vi "S2C_FORNAX_Proc_Commands.vi"(7 "VI_Ref":refnum<vi>, 8 "Error In":errorcluster, 10 "Settings":T1, 11 "Q-Ref":refnum<queue>) -> (0 "Error Out":errorcluster, 2 "Exit?":bool, 3 "Response":variant)   [LabVIEW 2015]
uses:
  S2C_FORNAX_Proc_Globals.vi
panel:
  out "Ref":refnum<k5>
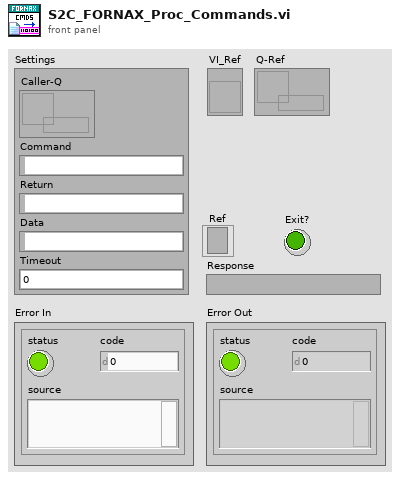
[diagram p1: front panel]
types:
  T1 = cluster{"Caller-Q":refnum<queue>, "Command":string, "Return":string, "Data":variant, "Timeout":dbl}
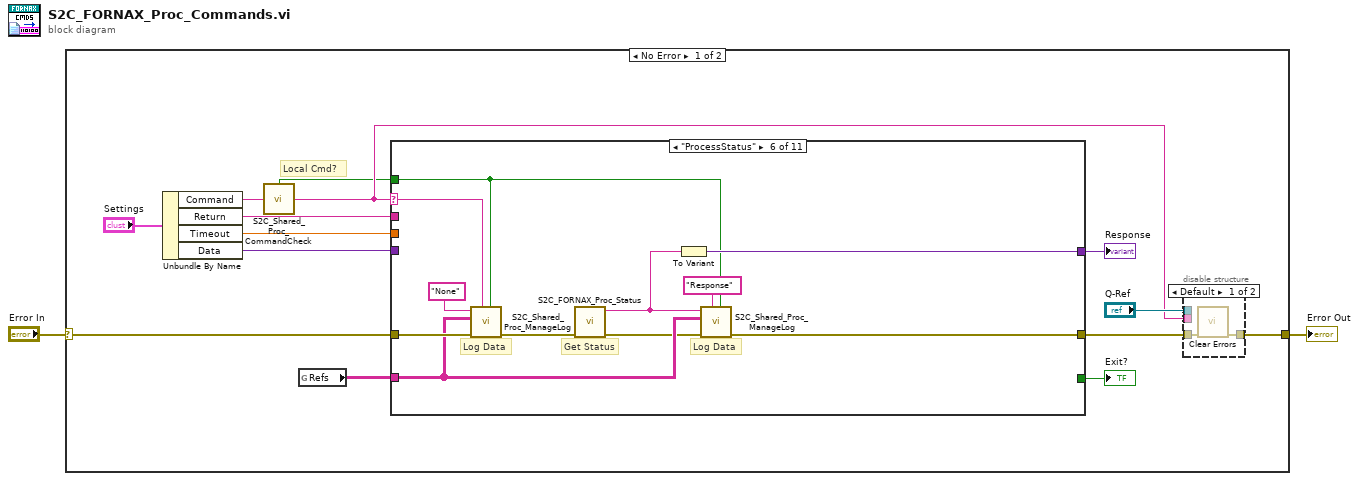
[diagram p0: block diagram]
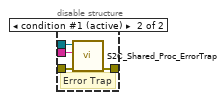
[diagram p2: hidden frame]
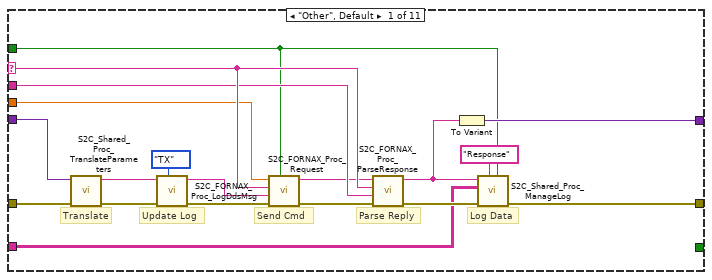
[diagram p3: hidden frame]
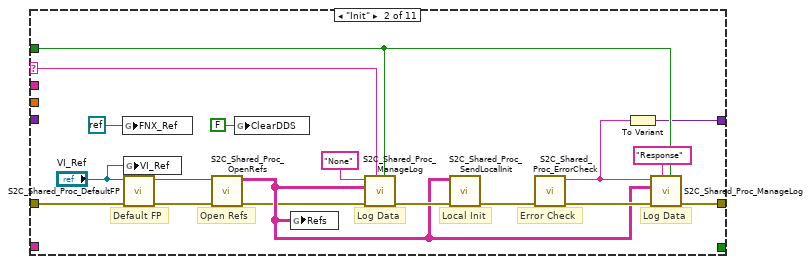
[diagram p4: hidden frame]
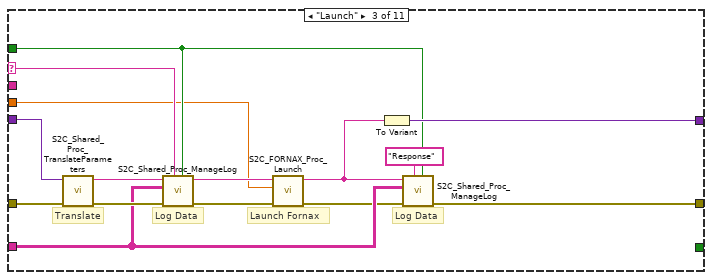
[diagram p5: hidden frame]
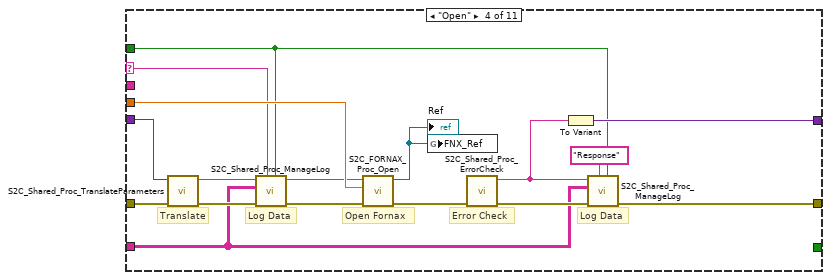
[diagram p6: hidden frame]
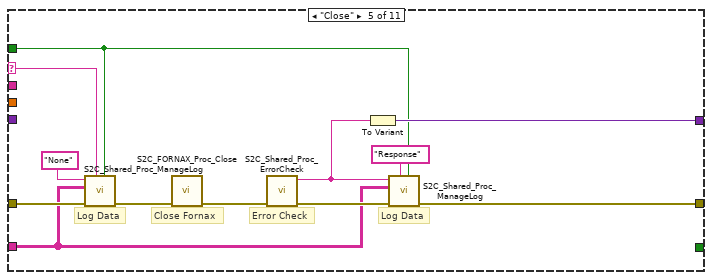
[diagram p7: hidden frame]
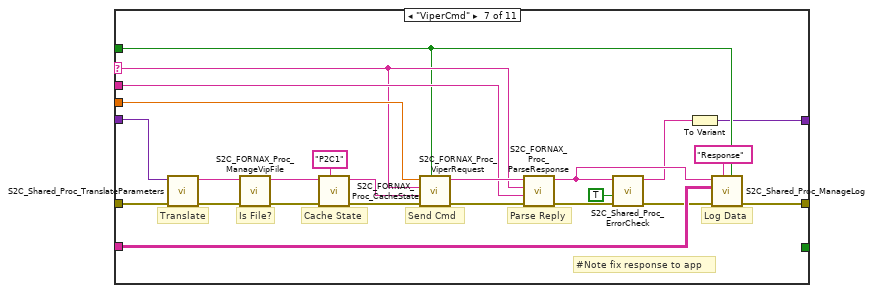
[diagram p8: hidden frame]
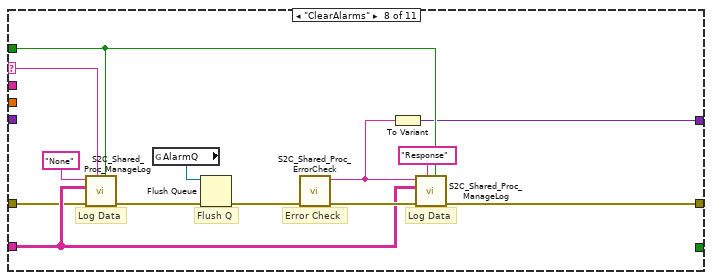
[diagram p9: hidden frame]
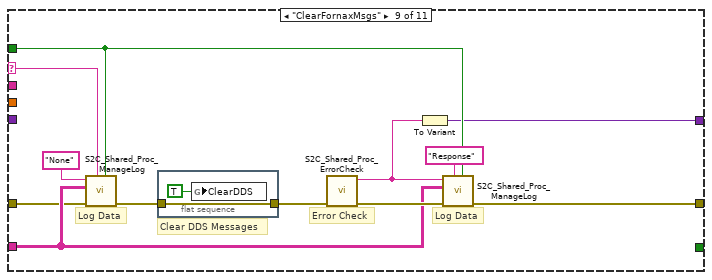
[diagram p10: hidden frame]
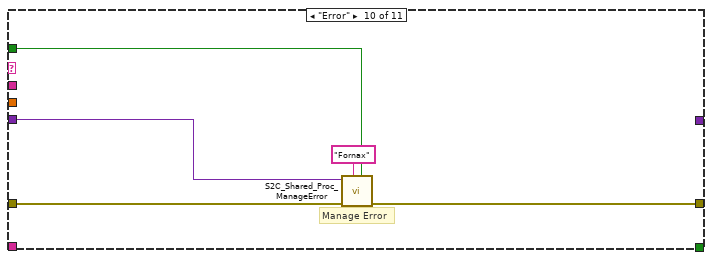
[diagram p11: hidden frame]
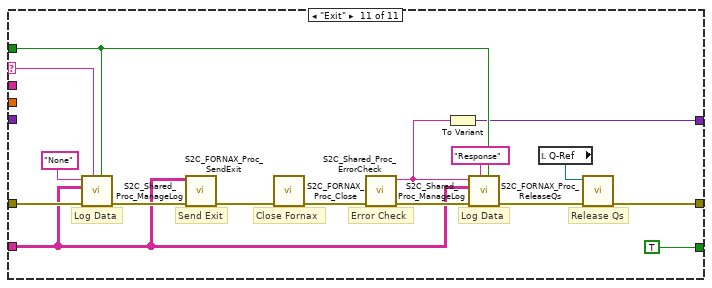
[diagram p12: hidden frame]
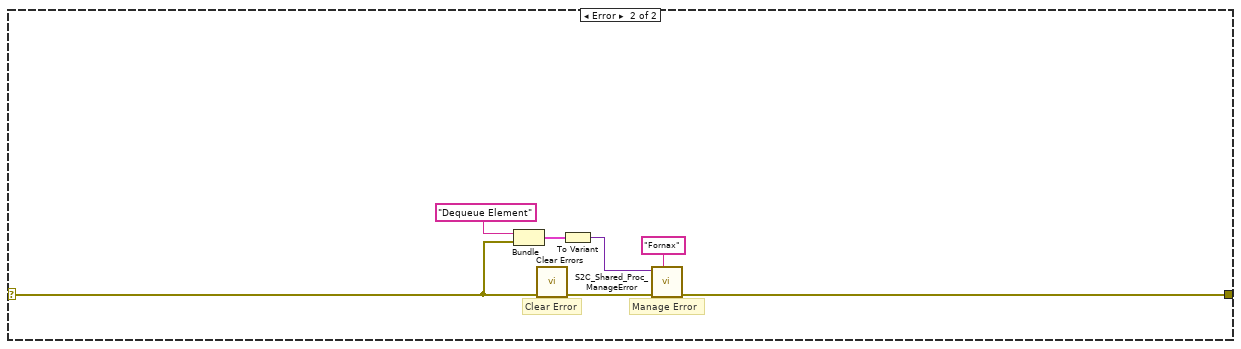
[diagram p13: hidden frame]
diagram:
  n1 = case shown="No Error" "Error In" {
    selector: "Error In" -> [w16 w188]
    tunnel: [w6 w187] -> w1
    frame No Error {
      # "Local Cmd?"
      n2 = Unbundle By Name("Settings") -> ("Command"=w5:string, "Return"=w13:string, "Timeout"=w11:dbl, "Data"=w12:variant)
      n3 = call "S2C_Shared_Proc_CommandCheck.vi"("Cmd In"=w5) -> ("Local?"=w3:bool, "Cmd Out"=w4:string)  [unwired: 13 in]
      n4 = global read "S2C_FORNAX_Proc_Globals.vi" "Refs"() -> (w9:string[][])
      n5 = case shown="\"ProcessStatus\"" w4 {
        selector: w4 -> [w38 w55 w69 w80 w99 w112 w132 w148 w160 _ w182]
        tunnel: w16 -> [w39 w46 w68 w90 w100 w113 w128 w142 w154 w169 w183]
        tunnel: [w31 w58 w66 w86 w93 w108 w130 w151 w163 w168 w172] -> w7
        tunnel: [w41 w48 w74 w91 w103 w114 w129 w144 w156 _ w175] -> w15
        tunnel: w13 -> [w37 _ _ _ _ _ w133 _ _ _ _]
        tunnel: w12 -> [w40 _ w73 w89 _ _ w127 _ _ w167 _]
        tunnel: w11 -> [w36 _ w61 w87 _ _ w134 _ _ _ _]
        tunnel: w3 -> [w30 w56 w70 w79 w98 w111 w131 w149 w161 w166 w181]
        tunnel: [_ _ _ _ _ _ _ _ _ _ TRUE] -> w10
        tunnel: w9 -> [w23 _ w65 w77 w92 w107 w135 w143 w155 _ w174]
        frame "Other", Default {
          # "Send Cmd"
          # "Update Log"
          # "Log Data"
          # "Parse Reply"
          # "Translate"
          n6 = call "S2C_Shared_Proc_TranslateParameters.vi"("Error In"=w39, "Data"=w40) -> ("Error Out"=w28:errorcluster, "JSON Cluster"=w27:string)  [unwired: 8 in]
          n7 = call "S2C_FORNAX_Proc_LogDdsMsg.vi"("Direction"=enum16{"TX", "RX"}."TX", "Error In"=w28, "Msg In"=w27) -> ("Error Out"=w25:errorcluster, "Msg Out"=w26:string)  [unwired: 7 in]
          n8 = call "S2C_FORNAX_Proc_Request.vi"("Local?"=w30, "Error In"=w25, "CmdString"=w26, "Command"=w38, "Timeout"=w36) -> ("Error Out"=w35:errorcluster, "Response"=w34:string)  [unwired: 5 in]
          n9 = call "S2C_FORNAX_Proc_ParseResponse.vi"("Error In"=w35, "Return"=w37, "Command"=w38, "JSON Response"=w34) -> ("Error Out"=w32:errorcluster, "Response"=w29:string)  [unwired: 6 in]
          n10 = To Variant(anything=w29) -> (Variant=w41:variant)
          n11 = call "S2C_Shared_Proc_ManageLog.vi"("Local?"=w30, "Command"="Response", "Error In"=w32, "Refs"=w23, "Data In"=w29) -> ("Error Out"=w31:errorcluster)  [unwired: 5 in, 1 out]
        }
        frame "Init" {
          # "Default FP"
          # "Local Init"
          # "Log Data"
          # "Error Check"
          # "Log Data"
          # "Open Refs"
          n12 = global write "S2C_FORNAX_Proc_Globals.vi" "FNX_Ref"(refnum<k0> refnum) -> ()
          n13 = global write "S2C_FORNAX_Proc_Globals.vi" "VI_Ref"("VI_Ref") -> ()
          n14 = call "S2C_Shared_Proc_DefaultFP.vi"("Error In"=w46, "VI_Ref In"="VI_Ref") -> ("Error Out"=w45:errorcluster, "VI_Ref Out"=w44:refnum<vi>)  [unwired: 8 in]
          n15 = call "S2C_Shared_Proc_OpenRefs.vi"("Error In"=w45, "VI_Ref"=w44) -> ("Error Out"=w47:errorcluster, "Refs"=w50:string[][])  [unwired: 8 in]
          n16 = global write "S2C_FORNAX_Proc_Globals.vi" "ClearDDS"(FALSE ("ClearDDS")) -> ()
          n17 = global write "S2C_FORNAX_Proc_Globals.vi" "Refs"(w50) -> ()
          n18 = call "S2C_Shared_Proc_ManageLog.vi"("Local?"=w56, "Command"=w55, "Error In"=w47, "Refs"=w50, "Data In"="None") -> ("Error Out"=w52:errorcluster)  [unwired: 5 in, 1 out]
          n19 = call "S2C_Shared_Proc_SendLocalInit.vi"("Error In"=w52, "Refs"=w50) -> ("Error Out"=w51:errorcluster)  [unwired: 9 in]
          n20 = call "S2C_Shared_Proc_ErrorCheck.vi"("Error In"=w51) -> ("Error Out"=w57:errorcluster, "Status"=w49:string)  [unwired: 9 in]
          n21 = To Variant(anything=w49) -> (Variant=w48:variant)
          n22 = call "S2C_Shared_Proc_ManageLog.vi"("Local?"=w56, "Command"="Response", "Error In"=w57, "Refs"=w50, "Data In"=w49) -> ("Error Out"=w58:errorcluster)  [unwired: 5 in, 1 out]
        }
        frame "Launch" {
          # "Launch Fornax"
          # "Log Data"
          # "Log Data"
          # "Translate"
          n23 = call "S2C_Shared_Proc_TranslateParameters.vi"("Error In"=w68, "Data"=w73) -> ("Error Out"=w72:errorcluster, "JSON Cluster"=w71:string)  [unwired: 8 in]
          n24 = call "S2C_Shared_Proc_ManageLog.vi"("Local?"=w70, "Command"=w69, "Error In"=w72, "Refs"=w65, "Data In"=w71) -> ("Error Out"=w64:errorcluster, "Data Out"=w62:string)  [unwired: 5 in]
          n25 = call "S2C_FORNAX_Proc_Launch.vi"("Error In"=w64, "Timeout"=w61, "Data"=w62) -> ("Error Out"=w63:errorcluster, "Result"=w60:string)  [unwired: 7 in]
          n26 = To Variant(anything=w60) -> (Variant=w74:variant)
          n27 = call "S2C_Shared_Proc_ManageLog.vi"("Local?"=w70, "Command"="Response", "Error In"=w63, "Refs"=w65, "Data In"=w60) -> ("Error Out"=w66:errorcluster)  [unwired: 5 in, 1 out]
        }
        frame "Open" {
          # "Open Fornax"
          # "Log Data"
          # "Error Check"
          # "Log Data"
          # "Translate"
          n28 = call "S2C_Shared_Proc_TranslateParameters.vi"("Error In"=w90, "Data"=w89) -> ("Error Out"=w82:errorcluster, "JSON Cluster"=w81:string)  [unwired: 8 in]
          n29 = call "S2C_Shared_Proc_ManageLog.vi"("Local?"=w79, "Command"=w80, "Error In"=w82, "Refs"=w77, "Data In"=w81) -> ("Error Out"=w75:errorcluster, "Data Out"=w76:string)  [unwired: 5 in]
          n30 = call "S2C_FORNAX_Proc_Open.vi"("Error In"=w75, "Timeout"=w87, "Data"=w76) -> ("Error Out"=w85:errorcluster, "FXN_Ref"=w88:refnum<k5>)  [unwired: 7 in]
          "Ref" <- w88
          n31 = global write "S2C_FORNAX_Proc_Globals.vi" "FNX_Ref"(w88) -> ()
          n32 = call "S2C_Shared_Proc_ErrorCheck.vi"("Error In"=w85) -> ("Error Out"=w84:errorcluster, "Status"=w83:string)  [unwired: 9 in]
          n33 = To Variant(anything=w83) -> (Variant=w91:variant)
          n34 = call "S2C_Shared_Proc_ManageLog.vi"("Local?"=w79, "Command"="Response", "Error In"=w84, "Refs"=w77, "Data In"=w83) -> ("Error Out"=w86:errorcluster)  [unwired: 5 in, 1 out]
        }
        frame "Close" {
          # "Log Data"
          # "Error Check"
          # "Log Data"
          # "Close Fornax"
          n35 = call "S2C_Shared_Proc_ManageLog.vi"("Local?"=w98, "Command"=w99, "Error In"=w100, "Refs"=w92, "Data In"="None") -> ("Error Out"=w96:errorcluster)  [unwired: 5 in, 1 out]
          n36 = call "S2C_FORNAX_Proc_Close.vi"("Error In"=w96) -> ("Error Out"=w102:errorcluster)  [unwired: 10 in]
          n37 = call "S2C_Shared_Proc_ErrorCheck.vi"("Error In"=w102) -> ("Error Out"=w94:errorcluster, "Status"=w101:string)  [unwired: 9 in]
          n38 = To Variant(anything=w101) -> (Variant=w103:variant)
          n39 = call "S2C_Shared_Proc_ManageLog.vi"("Local?"=w98, "Command"="Response", "Error In"=w94, "Refs"=w92, "Data In"=w101) -> ("Error Out"=w93:errorcluster)  [unwired: 5 in, 1 out]
        }
        frame "ProcessStatus" {
          # "Get Status"
          # "Log Data"
          # "Log Data"
          n40 = call "S2C_Shared_Proc_ManageLog.vi"("Local?"=w111, "Command"=w112, "Error In"=w113, "Refs"=w107, "Data In"="None") -> ("Error Out"=w106:errorcluster)  [unwired: 5 in, 1 out]
          n41 = call "S2C_FORNAX_Proc_Status.vi"("Error In"=w106) -> ("Error Out"=w104:errorcluster, "Response"=w105:string)  [unwired: 9 in]
          n42 = To Variant(anything=w105) -> (Variant=w114:variant)
          n43 = call "S2C_Shared_Proc_ManageLog.vi"("Local?"=w111, "Command"="Response", "Error In"=w104, "Refs"=w107, "Data In"=w105) -> ("Error Out"=w108:errorcluster)  [unwired: 5 in, 1 out]
        }
        frame "ViperCmd" {
          # "Cache State"
          # "Send Cmd"
          # "Is File?"
          # "Translate"
          # "#Note fix response to app"
          # "Log Data"
          # "Parse Reply"
          n44 = call "S2C_Shared_Proc_TranslateParameters.vi"("Error In"=w128, "Data"=w127) -> ("Error Out"=w124:errorcluster, "JSON Cluster"=w122:string)  [unwired: 8 in]
          n45 = call "S2C_FORNAX_Proc_ManageVipFile.vi"("Error In"=w124, "Data In"=w122) -> ("Error Out"=w123:errorcluster, "Data Out"=w121:string)  [unwired: 8 in]
          n46 = call "S2C_FORNAX_Proc_CacheState.vi"("Label"="P2C1", "Error In"=w123, "Data In"=w121) -> ("Error Out"=w120:errorcluster, "Data Out"=w119:string)  [unwired: 7 in]
          n47 = call "S2C_FORNAX_Proc_ViperRequest.vi"("Local?"=w131, "Error In"=w120, "CmdString"=w119, "Command"=w132, "Timeout"=w134) -> ("Error Out"=w138:errorcluster, "Response"=w137:string)  [unwired: 5 in]
          n48 = call "S2C_FORNAX_Proc_ParseResponse.vi"("Error In"=w138, "Return"=w133, "Command"=w132, "JSON Response"=w137) -> ("Error Out"=w126:errorcluster, "Response"=w117:string)  [unwired: 6 in]
          n49 = call "S2C_Shared_Proc_ErrorCheck.vi"("Error In"=w126, "ExpReply?"=TRUE, "Reply Text"=w117) -> ("Error Out"=w125:errorcluster, "Status"=w115:string)  [unwired: 7 in]
          n50 = To Variant(anything=w115) -> (Variant=w129:variant)
          n51 = call "S2C_Shared_Proc_ManageLog.vi"("Local?"=w131, "Command"="Response", "Error In"=w125, "Refs"=w135, "Data In"=w117) -> ("Error Out"=w130:errorcluster)  [unwired: 5 in, 1 out]
        }
        frame "ClearAlarms" {
          # "Flush Q"
          # "Log Data"
          # "Error Check"
          # "Log Data"
          n52 = call "S2C_Shared_Proc_ManageLog.vi"("Local?"=w149, "Command"=w148, "Error In"=w142, "Refs"=w143, "Data In"="None") -> ("Error Out"=w141:errorcluster)  [unwired: 5 in, 1 out]
          n53 = global read "S2C_FORNAX_Proc_Globals.vi" "AlarmQ"() -> (w139:refnum<queue>)
          n54 = Flush Queue(queue=w139, error in (no error)=w141) -> (error out=w140:errorcluster)  [unwired: 2 out]
          n55 = call "S2C_Shared_Proc_ErrorCheck.vi"("Error In"=w140) -> ("Error Out"=w150:errorcluster, "Status"=w145:string)  [unwired: 9 in]
          n56 = To Variant(anything=w145) -> (Variant=w144:variant)
          n57 = call "S2C_Shared_Proc_ManageLog.vi"("Local?"=w149, "Command"="Response", "Error In"=w150, "Refs"=w143, "Data In"=w145) -> ("Error Out"=w151:errorcluster)  [unwired: 5 in, 1 out]
        }
        frame "ClearFornaxMsgs" {
          # "Clear DDS Messages"
          # "Log Data"
          # "Error Check"
          # "Log Data"
          n58 = call "S2C_Shared_Proc_ManageLog.vi"("Local?"=w161, "Command"=w160, "Error In"=w154, "Refs"=w155, "Data In"="None") -> ("Error Out"=w153:errorcluster)  [unwired: 5 in, 1 out]
          n59 = flat-sequence {
            tunnel: w153 -> [w164]
            tunnel: [w164] -> w152
            frame #0 {
              n60 = global write "S2C_FORNAX_Proc_Globals.vi" "ClearDDS"(TRUE ("ClearDDS")) -> ()
            }
          }
          n61 = call "S2C_Shared_Proc_ErrorCheck.vi"("Error In"=w152) -> ("Error Out"=w162:errorcluster, "Status"=w157:string)  [unwired: 9 in]
          n62 = To Variant(anything=w157) -> (Variant=w156:variant)
          n63 = call "S2C_Shared_Proc_ManageLog.vi"("Local?"=w161, "Command"="Response", "Error In"=w162, "Refs"=w155, "Data In"=w157) -> ("Error Out"=w163:errorcluster)  [unwired: 5 in, 1 out]
        }
        frame "Error" {
          # "Manage Error"
          n64 = call "S2C_Shared_Proc_ManageError.vi"("Local?"=w166, "Process"="Fornax", "Error In"=w169, "Data"=w167) -> ("Error Out"=w168:errorcluster)  [unwired: 7 in]
        }
        frame "Exit" {
          # "Release Qs"
          # "Send Exit"
          # "Log Data"
          # "Error Check"
          # "Close Fornax"
          # "Log Data"
          n65 = call "S2C_Shared_Proc_ManageLog.vi"("Local?"=w181, "Command"=w182, "Error In"=w183, "Refs"=w174, "Data In"="None") -> ("Error Out"=w178:errorcluster)  [unwired: 5 in, 1 out]
          n66 = call "S2C_FORNAX_Proc_SendExit.vi"("Error In"=w178, "Refs"=w174) -> ("Error Out"=w177:errorcluster)  [unwired: 9 in]
          n67 = call "S2C_FORNAX_Proc_Close.vi"("Error In"=w177) -> ("Error Out"=w185:errorcluster)  [unwired: 10 in]
          n68 = call "S2C_Shared_Proc_ErrorCheck.vi"("Error In"=w185) -> ("Error Out"=w184:errorcluster, "Status"=w176:string)  [unwired: 9 in]
          n69 = To Variant(anything=w176) -> (Variant=w175:variant)
          n70 = call "S2C_Shared_Proc_ManageLog.vi"("Local?"=w181, "Command"="Response", "Error In"=w184, "Refs"=w174, "Data In"=w176) -> ("Error Out"=w173:errorcluster)  [unwired: 5 in, 1 out]
          n71 = local read "Q-Ref"() -> (w171:refnum<queue>)
          n72 = call "S2C_FORNAX_Proc_ReleaseQs.vi"("Error In"=w173, "Q-Ref"=w171) -> ("Error Out"=w172:errorcluster)  [unwired: 9 in]
        }
      }
      "Response" <- w15
      "Exit?" <- w10
      n73 = disable-structure shown="Default" {
        disable-tunnel: w7 -> [w18 w22]
        disable-tunnel: [w17 w21] -> w6
        disable-tunnel: w4 -> [_ w20]
        disable-tunnel: "Q-Ref" -> [_ w19]
        frame condition #0 {
          n74 = call <vilib>:"Clear Errors.vi"("error in (no error)"=w18) -> ("error out"=w17:errorcluster)  [unwired: 5 in, 1 out]
        }
        frame condition #1 (active) {
          # "Error Trap"
          n75 = call "S2C_Shared_Proc_ErrorTrap.vi"("Error In"=w22, "Command"=w20, "Q-Ref"=w19) -> ("Error Out"=w21:errorcluster)  [unwired: 8 in]
        }
      }
    }
    frame Error {
      # "Clear Error"
      # "Manage Error"
      n76 = Bundle("Dequeue Element", "error IO"=w188) -> (w192:cluster{string, "error IO":errorcluster})  [unwired: 1 in]
      n77 = call <vilib>:"Clear Errors.vi"("error in (no error)"=w188) -> ("error out"=w189:errorcluster)  [unwired: 5 in, 1 out]
      n78 = To Variant(anything=w192) -> (Variant=w190:variant)
      n79 = call "S2C_Shared_Proc_ManageError.vi"("Process"="Fornax", "Error In"=w189, "Data"=w190) -> ("Error Out"=w187:errorcluster)  [unwired: 8 in]
    }
  }
  "Error Out" <- w1
